vi "Control Microphone.vi"(0 "Session Handle in":T1, 5 "Command":u8=176 format="%x", 11 "error in (no error)":errorcluster) -> (4 "Session Handle out":T1, 6 "Success?":bool, 8 "Error Code":string, 15 "error out":errorcluster)   [LabVIEW 2015, in "PAS.lvclass"]
uses:
  PAS.lvclass
  Typedefs/Session Handle.ctl
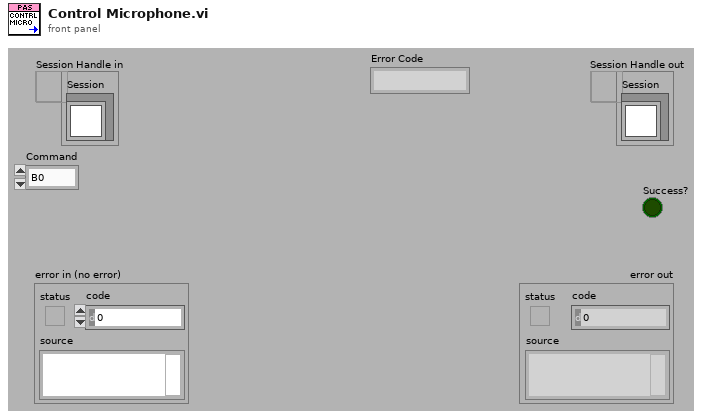
[diagram p1: front panel]
types:
  T1 = typedef "PAS.lvclass/Session Handle.ctl" = refnum<data-value>
  T2 = typedef "XNET Frame CAN.ctl" = cluster{"timestamp":timestamp, "payload":u8[], "identifier":u32, "type":T3, "extended?":bool, "echo?":bool}
  T3 = typedef "XNET Frame Type CAN.ctl" = u8
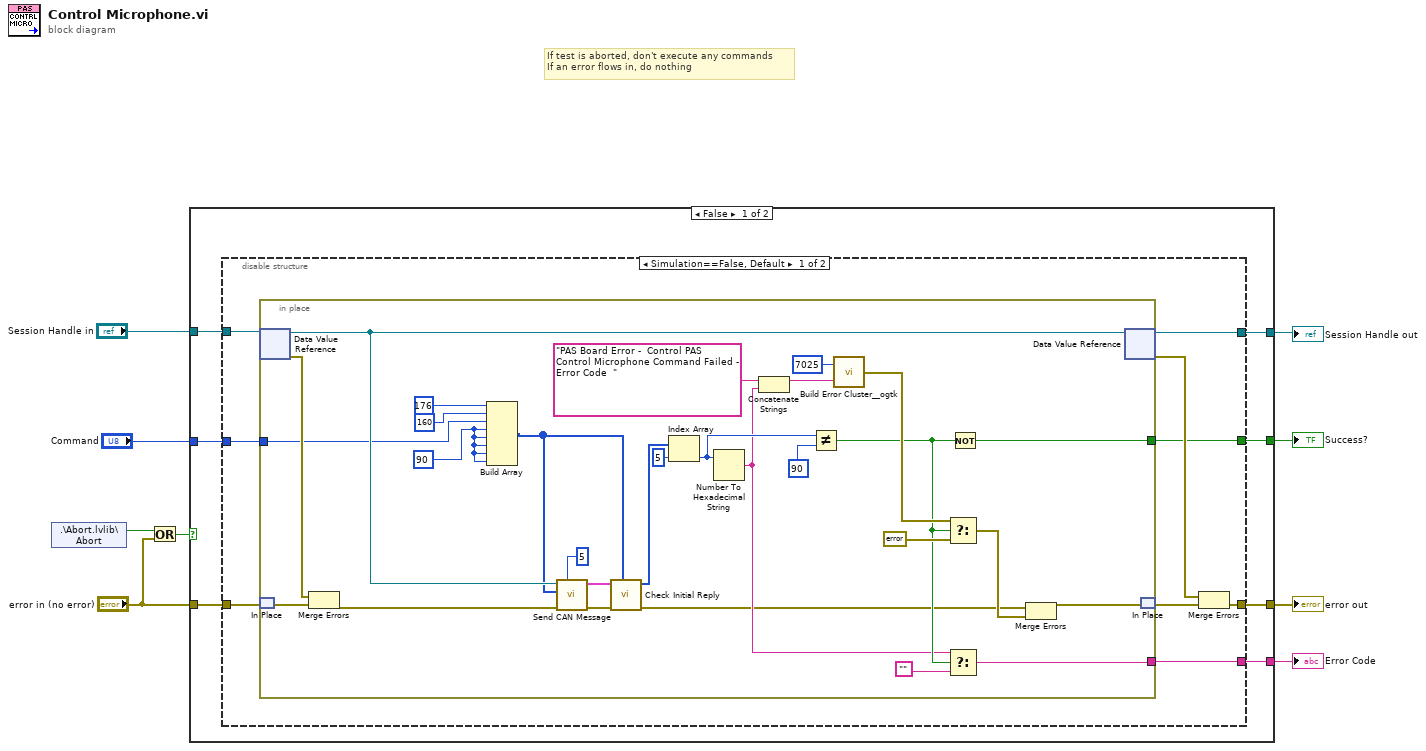
[diagram p0: block diagram]
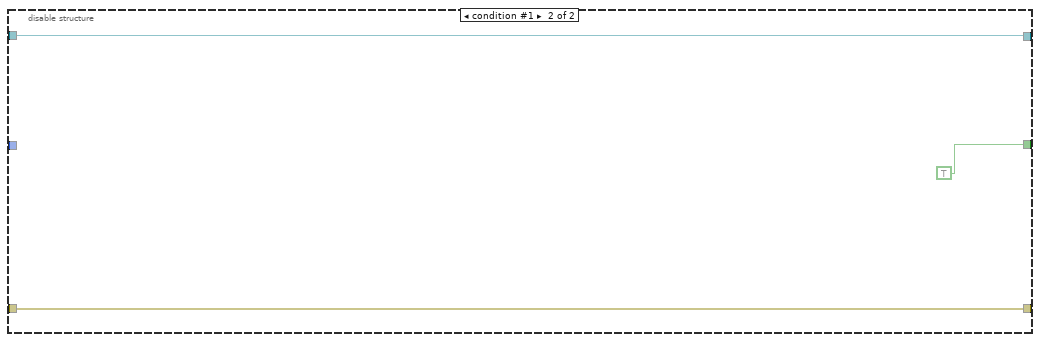
[diagram p2: hidden frame]
diagram:
  # "If test is aborted, don't execute any commands\nIf an error flows in, do nothing"
  n1 = shared-variable ".\\Abort.lvlib\\Abort"() -> (w6:bool)  [unwired: 1 in, 1 out]
  n2 = Or(x=w6, y="error in (no error)") -> (x .or. y?=w4:bool)
  n3 = case shown="False" w4 {
    tunnel: [w16 w59] -> w8
    tunnel: [w15 w58] -> w7
    tunnel: "Session Handle in" -> [w14 w59]
    tunnel: "error in (no error)" -> [w13 w58]
    tunnel: [w12 _] -> w3
    tunnel: [w11 _] -> w2
    tunnel: "Command" -> [w10 _]
    frame False {
      n4 = disable-structure shown="Simulation==False, Default" {
        disable-tunnel: [w25 w57] -> w16
        disable-tunnel: [w22 w56] -> w15
        disable-tunnel: w14 -> [w21 w57]
        disable-tunnel: w13 -> [w20 w56]
        disable-tunnel: [w19 TRUE] -> w12
        disable-tunnel: [w18 _] -> w11
        disable-tunnel: w10 -> [w17 _]
        frame condition #0 (active) {
          n5 = in-place {
            in-place-border: [w44] -> w19
            in-place-border: [w32] -> w18
            in-place-border: w17 -> [w28]
            w29 = u8 90 ("new element/subarray")
            n6 = in-place-dvr #1(w21) -> (w50:refnum<class "PAS.lvclass">, w53:errorcluster)
            n7 = in-place-match #2(w20) -> (w52:errorcluster)
            n8 = Merge Errors(w53, w52) -> (w51:errorcluster)
            n9 = Build Array(u8 176 ("new element/subarray"), u8 160 ("new element/subarray"), w28, w29, w29, w29, w29, w29) -> (w43:u8[])
            n10 = call "Send CAN Message.vi"("Number of Retries"=5, "error in (no error)"=w51, "payload"=w43, "Gas In"=w50) -> ("error out"=w27:errorcluster, "Reply"=w48:T2[])  [unwired: 5 in, 1 out]
            n11 = call "Check Initial Reply.vi"("Write Message"=w43, "error in (no error)"=w27, "Reply"=w48) -> ("error out"=w26:errorcluster, "Data Packet"=w42:u8[])  [unwired: 5 in, 2 out]
            n12 = Index Array(array=w42, index=5) -> (element=w38:u8)
            n13 = Number To Hexadecimal String(2:w38) -> (0:w33:string)  [unwired: 1 in]
            n14 = Concatenate Strings("PAS Board Error -  Control PAS Control Microphone Command Failed - Error Code  " ("string"), w33) -> (w39:string)
            n15 = Not Equal?(x=w38, y=u8 90 ("new element/subarray")) -> (x != y?=w34:bool)
            n16 = call <userlib>:"Build Error Cluster__ogtk.vi"("String to Prepend to source (\"\")"=w39, "code"=7025) -> ("error out"=w46:errorcluster)
            n17 = Select(t=w46, s=w34, f=errorcluster {"status"=FALSE, "code"=0, "source"=""}) -> (s? t:f=w36:errorcluster)
            n18 = Select(t=w33, s=w34, f="") -> (s? t:f=w32:string)
            n19 = Not(x=w34) -> (.not. x?=w44:bool)
            n20 = Merge Errors(w26, w36) -> (w54:errorcluster)
            n21 = in-place-dvr #1(w50) -> (w25:T1, w23:errorcluster)
            n22 = in-place-match #2(w54) -> (w24:errorcluster)
          }
          n23 = Merge Errors(w23, w24) -> (w22:errorcluster)
        }
        frame condition #1 {
        }
      }
    }
    frame True {
    }
  }
  "Session Handle out" <- w8
  "error out" <- w7
  "Success?" <- w3
  "Error Code" <- w2
